vi "Main.vi"() -> ()   [LabVIEW 2021]
panel:
  out "Booléen":bool
  out "Graphe":dbl[](graph)
  out "x+y":dbl
  in  "y":dbl
  in  "x":dbl
  in  "stop":bool
  # "hELLO Fabien"
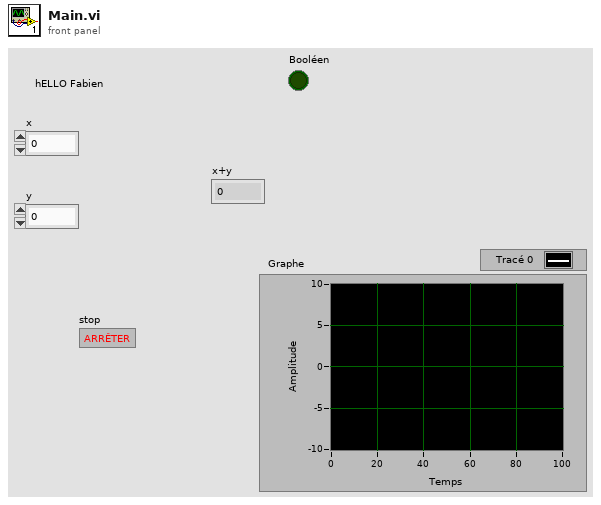
[diagram p1: front panel]
types:
  T1 = enum32{"invalid app kind", "Development System", "Run Time System", "Student Edition", "Embedded LabVIEW", "Evaluation", "Custom"}
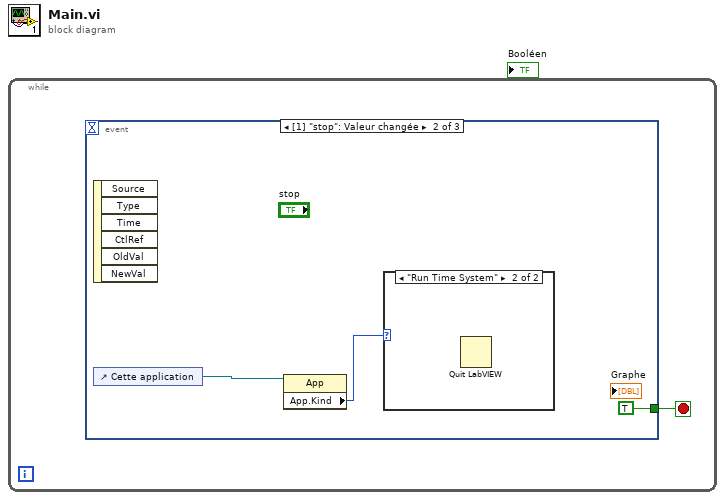
[diagram p0: block diagram]
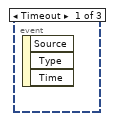
[diagram p2: hidden frame]
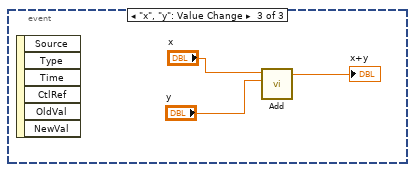
[diagram p4: hidden frame]
diagram:
  n1 = while {
    stop <- w1 stop-if-true
    n2 = event shown="[1] \"stop\": Valeur changée" {
      selector: _ -> [_ _ _]
      dyn-events: _ -> [_ _ _]
      timeout: _ -> [_ _ _]
      tunnel: [_ TRUE _] -> w1
      event Timeout {
        n3 = event-data() -> ()  [unwired: 1 in, 3 out]
      }
      event "stop": Value Change {
        n4 = event-data() -> ()  [unwired: 1 in, 6 out]
        n5 = control-ref of="Cette application"() -> (w3:refnum<vi>)
        n6 = property class="App"(reference=w3) -> ("App.Kind"=w2:T1)  [unwired: 1 in, 2 out]
        n7 = case shown="\"Run Time System\"" w2 {
          frame "invalid app kind", Default {
          }
          frame "Run Time System" {
            n8 = Quit LabVIEW() -> ()  [unwired: 1 in]
          }
        }
      }
      event "x", "y": Value Change {
        n9 = event-data() -> ()  [unwired: 1 in, 6 out]
        n10 = call "Add.vi"("y"="y", "x"="x") -> ("x+y"=→"x+y":dbl)  [unwired: 9 in]
      }
    }
  }
